vi "Generuj_start_event.vi"(8 "error in (no error)":errorcluster) -> (0 "error out":errorcluster, 3 "Event Registration Refnum out":refnum<event-registration>, 5 "user event out":refnum<user-event>)   [LabVIEW 2014]
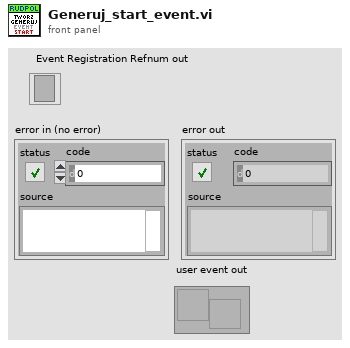
[diagram p1: front panel]
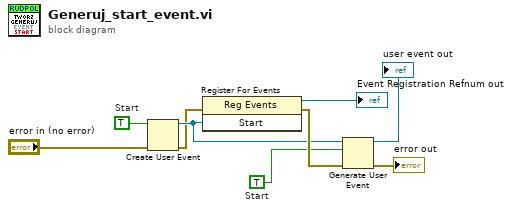
[diagram p0: block diagram]
diagram:
  w8 = TRUE  # Start
  w5 = TRUE  # Start
  n1 = Create User Event(user event datatype=w5, error in="error in (no error)") -> (user event=w7:refnum<user-event>, error out=w6:errorcluster)
  n2 = register-events(error in=w6, w7) -> (reference out=→"Event Registration Refnum out":refnum<event-registration>, error out=w9:errorcluster)  [unwired: 1 in]
  n3 = Generate User Event(user event=w7, event data cluster=w8, error in=w9) -> (user event out=→"user event out":refnum<user-event>, error out=→"error out":errorcluster)  [unwired: 1 in]
